vi "Get Number Text.vi"(8 "error in (no error)":errorcluster, 10 "Offset":i32, 11 "JSON":string) -> (0 "error out":errorcluster, 1 "Offset past match":i32, 2 "Number Text":string, 4 "JSON Value Type":T1)   [LabVIEW 2017, in "JSONtext.lvlib"]
uses:
  JSONtext.lvlib
  JSON Value Type.ctl
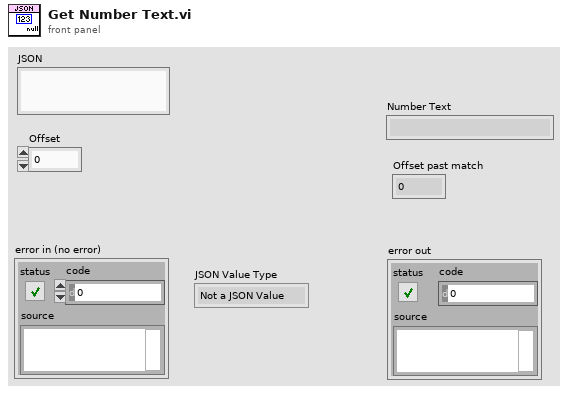
[diagram p1: front panel]
types:
  T1 = typedef "JSONtext.lvlib/JSON Value Type.ctl" = enum16{"Not a JSON Value", "JSON Object", "JSON Array", "String", "Number", "true", "false", "null"}
  T2 = typedef "JSONtext.lvlib/Parsing State.ctl" = enum16{"Parser Error", "Object", "Array", "String", "Number/Other", "Leading Whitespace", "Object end", "Array end", "Value end"}
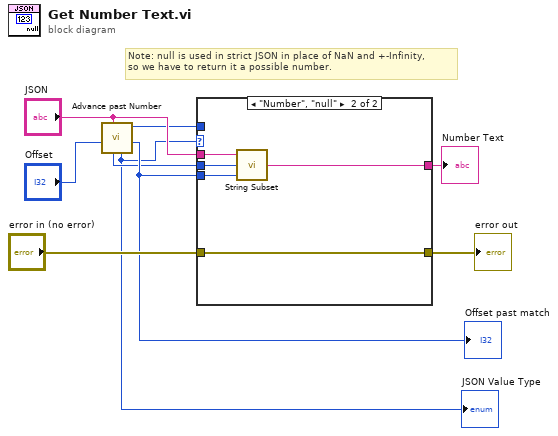
[diagram p0: block diagram]
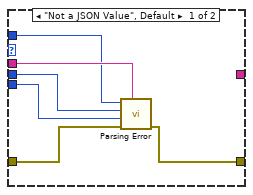
[diagram p2: hidden frame]
diagram:
  # "Note: null is used in strict JSON in place of NaN and +-Infinity,\nso we have to return it a possible number."
  n1 = call "Advance past Number.vi"("JSON"="JSON", "Offset (0)"="Offset") -> ("Offset past match"=w4:i32, "Parser State"=w1:T2, "JSON Value Type"=w2:T1, "Value start out"=w3:i32)  [unwired: 6 in]
  "Offset past match" <- w4
  "JSON Value Type" <- w2
  n2 = case shown="\"Number\", \"null\"" w2 {
    tunnel: "JSON" -> [w13 w20]
    tunnel: [w15 w16] -> w7
    tunnel: "error in (no error)" -> [w14 w16]
    tunnel: [_ w17] -> w5
    tunnel: w3 -> [w12 w19]
    tunnel: w4 -> [w11 w18]
    tunnel: w1 -> [w10 _]
    frame "Not a JSON Value", Default {
      n3 = call "Parsing Error.vi"("JSON"=w13, "error in (no error)"=w14, "Offset past match"=w11, "Value start"=w12, "State"=w10) -> ("error out"=w15:errorcluster)  [unwired: 6 in]
    }
    frame "Number", "null" {
      n4 = call "String Subset.vi"("Offset past End"=w18, "Start offset"=w19, "JSON"=w20) -> ("substring"=w17:string)  [unwired: 2 in]
    }
  }
  "error out" <- w7
  "Number Text" <- w5
